vi "Create&Start.vi"(8 "error in (no error)":errorcluster, 11 "XML config File Path":path=path "D:/work/Project support in lanzhou/OPCUA XML/xml/server config.xml") -> (0 "error out":errorcluster, 2 "Parse Errors":string, 3 "server endpoint URL":string, 4 "trusted client certfications":path[](array[path]))   [LabVIEW 2014, in "OPCUA Server(UtilityMode)(dev).lvlib"]
uses:
  OPCUA Server(UtilityMode)(dev).lvlib
  _op(server).ctl
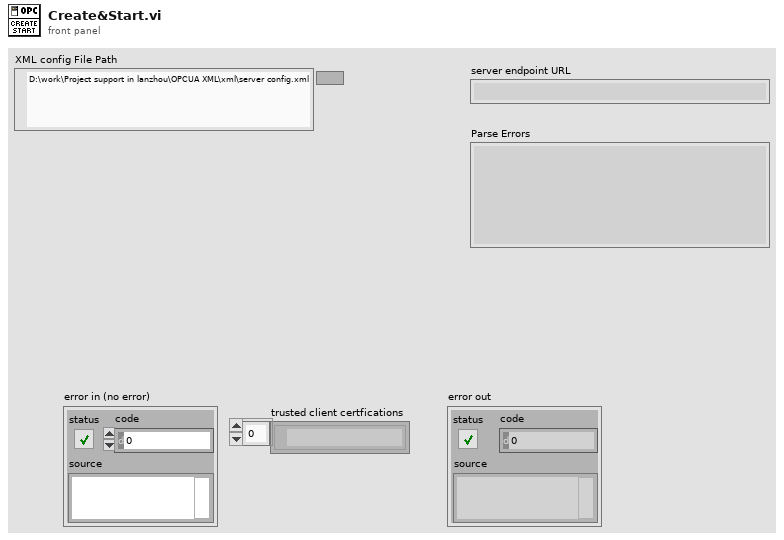
[diagram p1: front panel]
types:
  T1 = typedef "OPCUA Server(UtilityMode)(dev).lvlib/_op(server).ctl" = enum16{"Create Server", "Start Server", "Get Server Refnum", "Stop Server", "Close Server"}
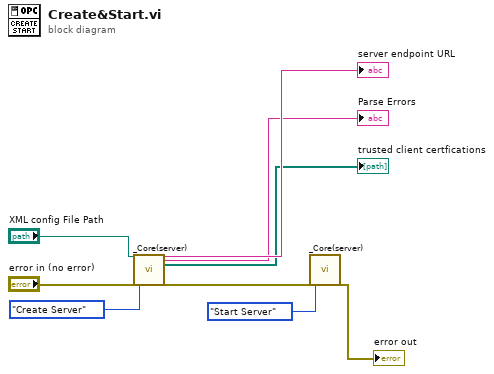
[diagram p0: block diagram]
diagram:
  n1 = call "_Core(server).vi"("XML config File Path"="XML config File Path", "error in (no error)"="error in (no error)", "Op"=_op(server)."Create Server") -> ("server endpoint URL"=→"server endpoint URL":string, "Parse Errors"=→"Parse Errors":string, "trusted client certfications"=→"trusted client certfications":path[], "error out"=w3:errorcluster)  [unwired: 20 in, 1 out]
  n2 = call "_Core(server).vi"("error in (no error)"=w3, "Op"=_op(server)."Start Server") -> ("error out"=→"error out":errorcluster)  [unwired: 21 in, 4 out]
